vi "Execute State Change Callback.vi"(8 "error in (no error)":errorcluster, 9 "Connection State":bool, 10 "Connection ID":string, 11 "EventConnectionCallback in":refnum<class "EventConnectionCallback.lvclass">) -> (0 "error out":errorcluster)   [LabVIEW 2019, in "EventConnectionCallback.lvclass"]
uses:
  <vilib>/gpm_packages/@cs/Network-interface/Examples/EventConnectionCallback/EventConnectionCallback.lvclass
  <vilib>/gpm_packages/@cs/Network-interface/Examples/EventConnectionCallback/ConnectionStateType.ctl
  <vilib>/gpm_packages/@cs/Network-interface/Examples/EventConnectionCallback/EventConnectionCallback.lvclass/EventConnectionCallback.ctl
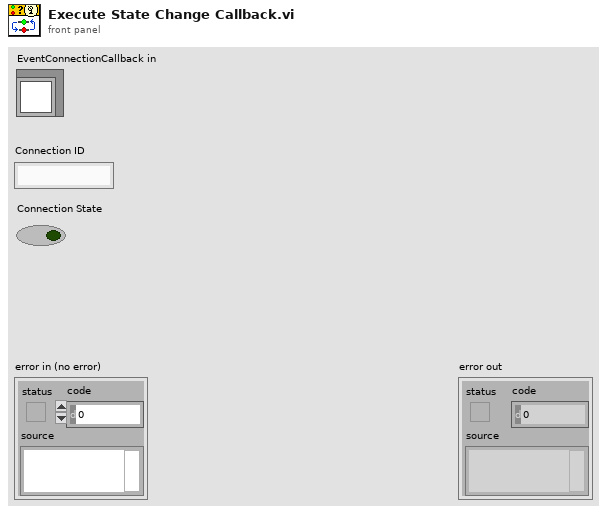
[diagram p1: front panel]
types:
  T1 = typedef "EventConnectionCallback.lvclass/ConnectionStateType.ctl" = cluster{"Connection ID":string, "State":bool}
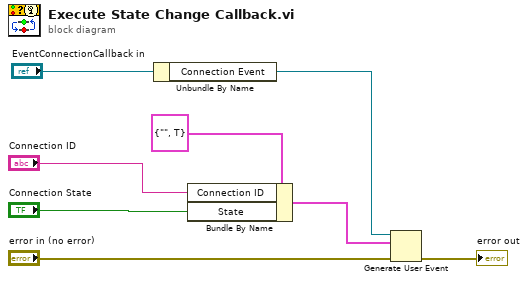
[diagram p0: block diagram]
diagram:
  n1 = Unbundle By Name("EventConnectionCallback in") -> ("Connection Event"=w2:refnum<user-event>)
  n2 = Bundle By Name(cluster=T1 {"Connection ID"="", "State"=TRUE}, "Connection ID"="Connection ID", "State"="Connection State") -> (w1:T1)
  n3 = Generate User Event(user event=w2, event data cluster=w1, error in="error in (no error)") -> (error out=→"error out":errorcluster)  [unwired: 1 in, 1 out]
